vi "Configure IO Type.vi"(0 "VISA resource name":refnum<visa-resource-name>, 1 "Number(0)":dbl, 2 "Type(0:OFFSta)":u16(ring) items=["OFFSta", "PSSTa", "INHLiv", "EXTTrig", "SYON", "SYOFF", "INHLat", "IORD", "IOWR", "PSCLear", "PWＭ", "TOUT"], 3 "error in (no error)":errorcluster) -> (7 "VISA resource name out":refnum<visa-resource-name>, 10 "error out":errorcluster)   [LabVIEW 2015, in "IT6000C.lvlib"]
doc: "This command sets the IO type, which can usually be set to the first function and three second functions (IORD, IOWR, and PWM). The default first functions of the seven IO ports are: PSCLear, PASSta, OFFSta, EXTTrig, INHLiv (INHLat), SYON, SYOFF.\n\n\n<b>Type</b>\n0:OFFSta\n1:PSSTa\n2:INHLiv\n3:EXTTrig\n4:SYON\n5:SYOFF\n6:INHLat\n7:IORD\n8:IOWR\n9:PSCLear\n10:PWM\n11:TOUT"
uses:
  <instrlib>/IT6000C/IT6000C.lvlib
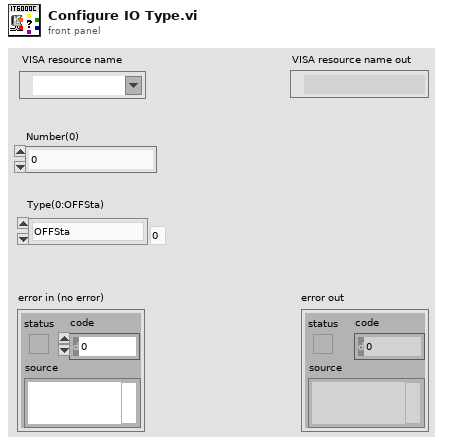
[diagram p1: front panel]
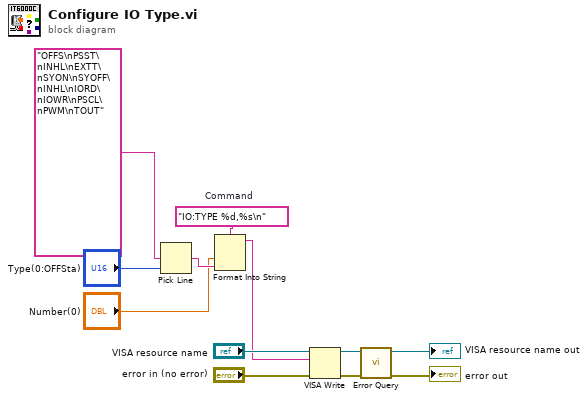
[diagram p0: block diagram]
diagram:
  w6 = "IO:TYPE %d,%s\n"  # Command
  n1 = Pick Line(multi-line string="OFFS\nPSST\nINHL\nEXTT\nSYON\nSYOFF\nINHL\nIORD\nIOWR\nPSCL\nPWM\nTOUT", line index="Type(0:OFFSta)") -> (output string=w2:string)  [unwired: 1 in]
  n2 = Format Into String(format string=w6, "Number(0)", w2) -> (resulting string=w5:string)  [unwired: 2 in, 1 out]
  n3 = VISA Write(VISA resource name="VISA resource name", write buffer=w5, error in (no error)="error in (no error)") -> (VISA resource name out=w9:refnum<visa-resource-name>, error out=w10:errorcluster)  [unwired: 1 out]
  n4 = call <instrlib>:"Error Query.vi"("error in (no error)"=w10, "VISA resource name"=w9) -> ("error out"=→"error out":errorcluster, "VISA resource name out"=→"VISA resource name out":refnum<visa-resource-name>)  [unwired: 6 in, 2 out]
